vi "Ephys.vi"() -> ()   [LabVIEW 2014]
uses:
  Electrophysiology/Electrophysiology.lvclass
  IntanElectrophysiology/IntanElectrophysiology.lvclass
  IntanElectrophysiology/IntanElectrophysiology.lvclass/IntanElectrophysiology.ctl
panel:
  in  "Base Path For Intan Task Files":path=path "c:/IntanTasks"
  in  "Intan Task":u16(ring)
  in  "Start":bool
  out "Stopped":bool
  in  "Link":bool
  in  "Audio":cluster{"Left":u16, "Right":u16} {"Right" items=["Electrode01"=0, "Electrode02"=1, "Electrode03"=2, "Electrode04"=3, "Electrode05"=4, "Electrode06"=5, "Electrode07"=6, "Electrode08"=7, "Electrode09"=8, "Electrode10"=9, "Electrode11"=10, "Electrode12"=11, "Electrode13"=12, "Electrode14"=13, "Electrode15"=14, "Electrode16"=15, "Electrode17"=16, "Electrode18"=17, "Electrode19"=18, "Electrode20"=19, "Electrode21"=20, "Electrode22"=21, "Electrode23"=22, "Electrode24"=23, "Electrode25"=24, "Electrode26"=25, "Electrode27"=26, "Electrode28"=27, "Electrode29"=28, "Electrode30"=29, "Electrode31"=30, "Electrode32"=31, "Electrode33"=32, "Electrode34"=33, "Electrode35"=34, "Electrode36"=35, "Electrode37"=36, "Electrode38"=37, "Electrode39"=38, "Electrode40"=39, "Electrode41"=40, "Electrode42"=41, "Electrode43"=42, "Electrode44"=43, "Electrode45"=44, "Electrode46"=45, "Electrode47"=46, "Electrode48"=47, "Electrode49"=48, "Electrode50"=49, "Electrode51"=50, "Electrode52"=51, "Electrode53"=52, "Electrode54"=53, "Electrode55"=54, "Electrode56"=55, "Electrode57"=56, "Electrode58"=57, "Electrode59"=58, "Electrode60"=59, "Electrode61"=60, "Electrode62"=61, "Electrode63"=62, "Electrode64"=63, "Electrode65"=64, "Electrode66"=65, "Electrode67"=66, "Electrode68"=67, "Electrode69"=68, "Electrode70"=69, "Electrode71"=70, "Electrode72"=71, "Electrode73"=72, "Electrode74"=73, "Electrode75"=74, "Electrode76"=75, "Electrode77"=76, "Electrode78"=77, "Electrode79"=78, "Electrode80"=79, "Electrode81"=80, "Electrode82"=81, "Electrode83"=82, "Electrode84"=83, "Electrode85"=84, "Electrode86"=85, "Electrode87"=86, "Electrode88"=87, "Electrode89"=88, "Electrode90"=89, "Electrode91"=90, "Electrode92"=91, "Electrode93"=92, "Electrode94"=93, "Electrode95"=94, "Electrode96"=95, "Gnd1"=96, "Gnd2"=97, "Gnd3"=98, "Gnd4"=99, "Photodiode"=102, "Ref1"=100, "Ref2"=101]; "Left" items=["Electrode01"=0, "Electrode02"=1, "Electrode03"=2, "Electrode04"=3, "Electrode05"=4, "Electrode06"=5, "Electrode07"=6, "Electrode08"=7, "Electrode09"=8, "Electrode10"=9, "Electrode11"=10, "Electrode12"=11, "Electrode13"=12, "Electrode14"=13, "Electrode15"=14, "Electrode16"=15, "Electrode17"=16, "Electrode18"=17, "Electrode19"=18, "Electrode20"=19, "Electrode21"=20, "Electrode22"=21, "Electrode23"=22, "Electrode24"=23, "Electrode25"=24, "Electrode26"=25, "Electrode27"=26, "Electrode28"=27, "Electrode29"=28, "Electrode30"=29, "Electrode31"=30, "Electrode32"=31, "Electrode33"=32, "Electrode34"=33, "Electrode35"=34, "Electrode36"=35, "Electrode37"=36, "Electrode38"=37, "Electrode39"=38, "Electrode40"=39, "Electrode41"=40, "Electrode42"=41, "Electrode43"=42, "Electrode44"=43, "Electrode45"=44, "Electrode46"=45, "Electrode47"=46, "Electrode48"=47, "Electrode49"=48, "Electrode50"=49, "Electrode51"=50, "Electrode52"=51, "Electrode53"=52, "Electrode54"=53, "Electrode55"=54, "Electrode56"=55, "Electrode57"=56, "Electrode58"=57, "Electrode59"=58, "Electrode60"=59, "Electrode61"=60, "Electrode62"=61, "Electrode63"=62, "Electrode64"=63, "Electrode65"=64, "Electrode66"=65, "Electrode67"=66, "Electrode68"=67, "Electrode69"=68, "Electrode70"=69, "Electrode71"=70, "Electrode72"=71, "Electrode73"=72, "Electrode74"=73, "Electrode75"=74, "Electrode76"=75, "Electrode77"=76, "Electrode78"=77, "Electrode79"=78, "Electrode80"=79, "Electrode81"=80, "Electrode82"=81, "Electrode83"=82, "Electrode84"=83, "Electrode85"=84, "Electrode86"=85, "Electrode87"=86, "Electrode88"=87, "Electrode89"=88, "Electrode90"=89, "Electrode91"=90, "Electrode92"=91, "Electrode93"=92, "Electrode94"=93, "Electrode95"=94, "Electrode96"=95, "Gnd1"=96, "Gnd2"=97, "Gnd3"=98, "Gnd4"=99, "Photodiode"=102, "Ref1"=100, "Ref2"=101]}
  in  "Volume":dbl(slide)=1.0608183551394462e-08 scale=1e-11..1e-05
  in  "Play":bool
  out "Streaming":bool
  out "Writing Error":bool
  in  "Record":bool=TRUE
  out "Writing Backlog":i32
  in  "NI Recording Task":refnum<k21>="All4498"
  out "MSamples":dbl
  in  "Stop":bool
  # "Audio"
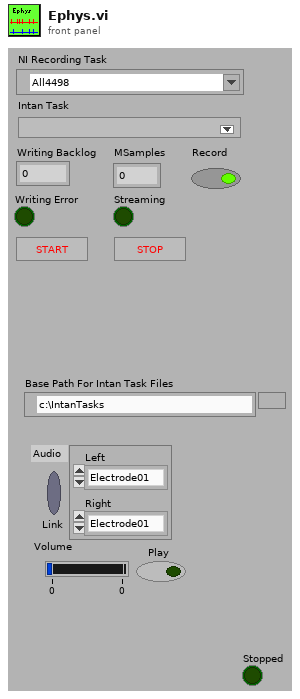
[diagram p1: front panel]
types:
  T1 = enum8{"Enabled", "Disabled", "Disabled and Grayed Out"}
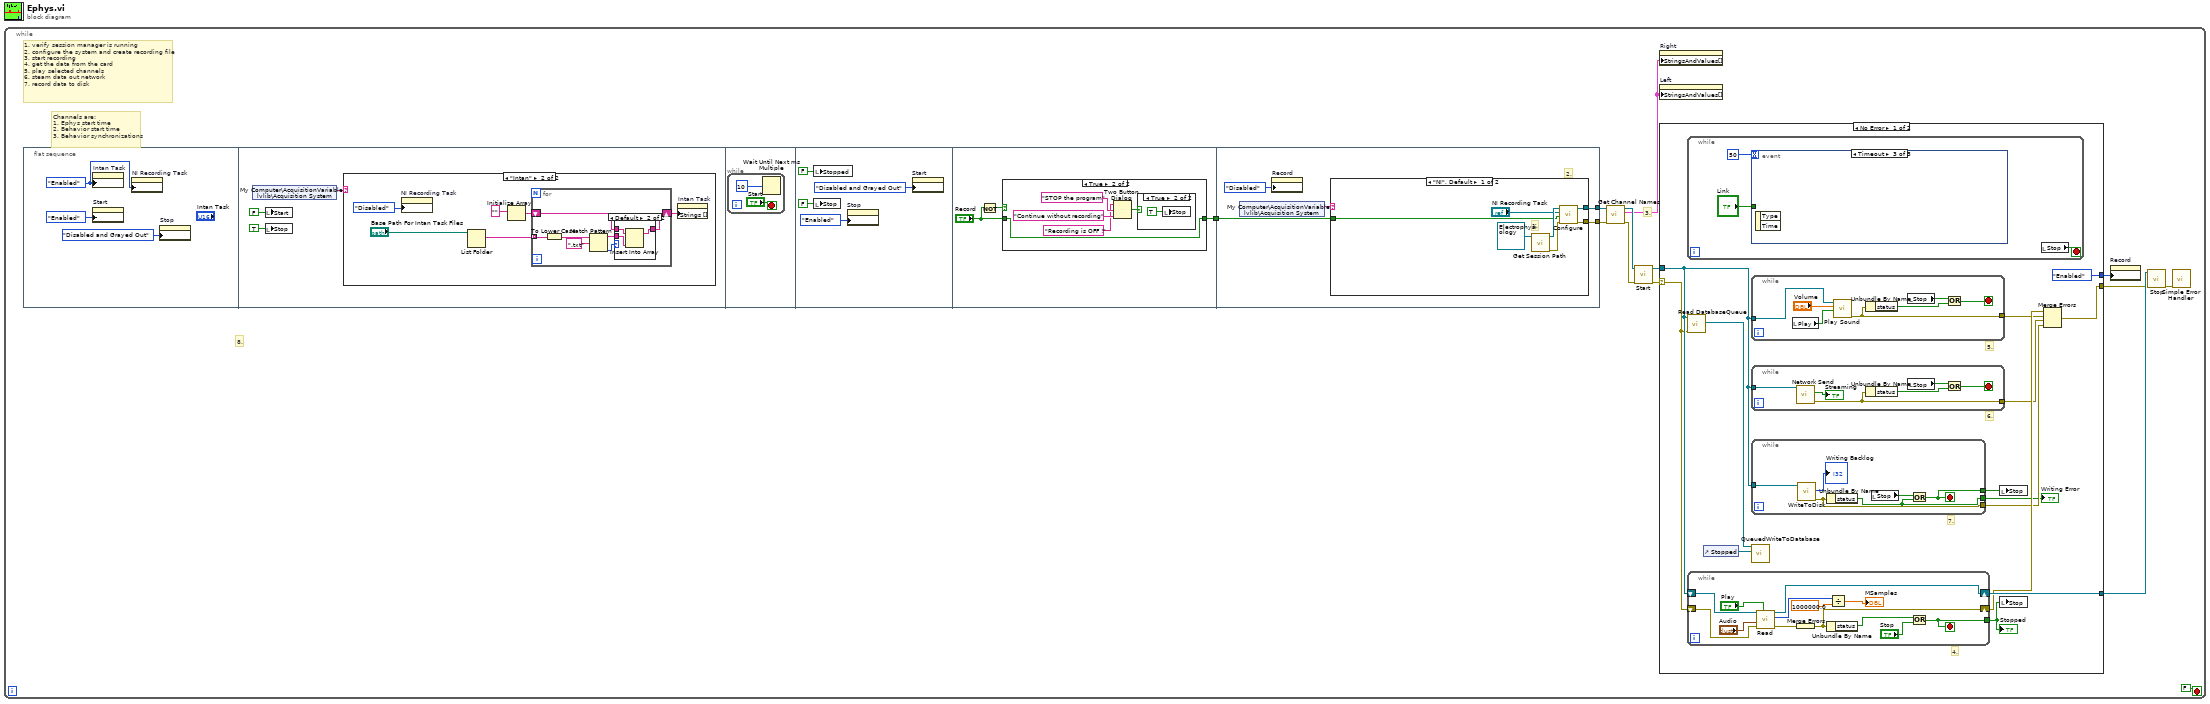
[diagram p0: block diagram]
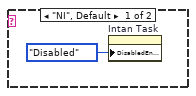
[diagram p2: hidden frame]
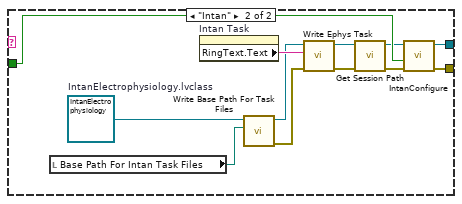
[diagram p6: hidden frame]
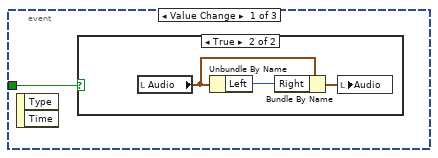
[diagram p7: hidden frame]
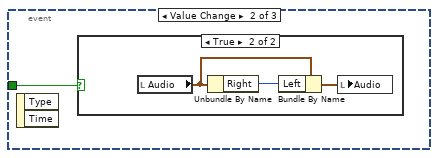
[diagram p9: hidden frame]
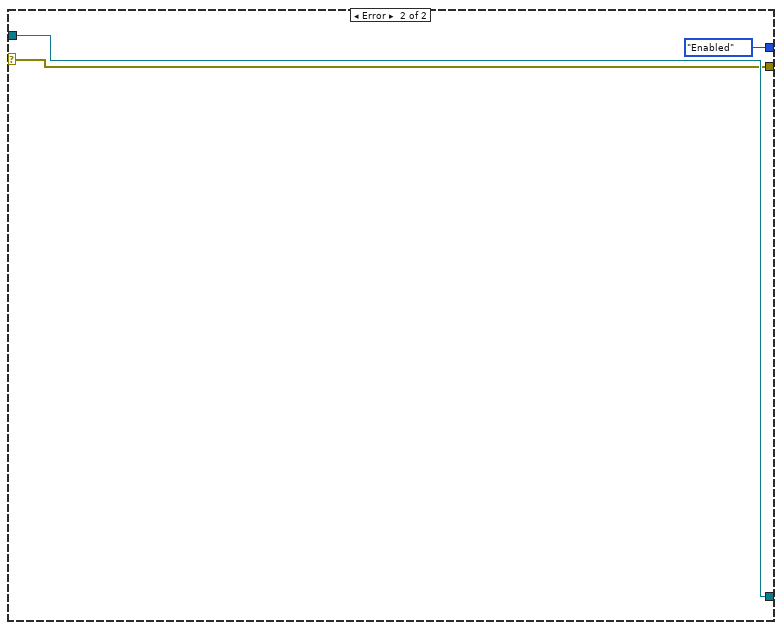
[diagram p11: hidden frame]
diagram:
  n1 = while {
    stop <- FALSE stop-if-true
    # "8."
    # "1. verify session manager is running\n2. configure the system and create recording file\n3. start recording\n4. get the data from the card\n5. play selected channels\n6. steam data out network\n7. record data to disk"
    # "3."
    # "Channels are:\n1. Ephys start time\n2. Behavior start time\n3. Behavior synchronizations"
    n2 = flat-sequence {
      tunnel: [w44] -> w13
      tunnel: [w58] -> w1
      tunnel: w13 -> [w56]
      tunnel: [w55] -> w2
      frame #0 {
        w16 = T1."Enabled" ("Disabled")
        n3 = property on="Intan Task" class="Ring (strict)"("DisabledEnum"=w16) -> ()  [unwired: 2 in, 2 out]
        n4 = property on="Start" class="Bool (strict)"("DisabledEnum"=T1."Enabled" ("Disabled")) -> ()  [unwired: 2 in, 2 out]
        n5 = property on="NI Recording Task" class="DAQmxName (strict)"("DisabledEnum"=w16) -> ()  [unwired: 2 in, 2 out]
        n6 = property on="Stop" class="Bool (strict)"("DisabledEnum"=T1."Disabled and Grayed Out" ("Disabled")) -> ()  [unwired: 2 in, 2 out]
      }
      frame #1 {
        n7 = shared-variable "My Computer\\AcquisitionVariables.lvlib\\Acquisition System"() -> (w17:string)  [unwired: 1 in, 1 out]
        n8 = local write "Start"(FALSE ("Start")) -> ()
        n9 = local write "Stop"(TRUE ("Stop")) -> ()
        n10 = case shown="\"Intan\"" w17 {
          frame "NI", Default {
            n11 = property on="Intan Task" class="Ring (strict)"("DisabledEnum"=T1."Disabled" ("Disabled")) -> ()  [unwired: 2 in, 2 out]
          }
          frame "Intan" {
            n12 = property on="NI Recording Task" class="DAQmxName (strict)"("DisabledEnum"=T1."Disabled" ("Disabled")) -> ()  [unwired: 2 in, 2 out]
            n13 = List Folder(path="Base Path For Intan Task Files") -> (filenames=w24:string[])  [unwired: 3 in, 3 out]
            n14 = Initialize Array("") -> (w22:string[])  [unwired: 1 in]
            n15 = for {
              tunnel: w24 -> [w33] mode=indexing
              shift-right: [w29] -> w21
              shift-left: w22 -> [w28]
              n16 = To Lower Case(string=w33) -> (all lower case string=w32:string)
              n17 = Match Pattern(string=w32, regular expression=".txt") -> (before substring=w27:string, offset past match=w30:i32)  [unwired: 1 in, 2 out]
              n18 = case shown="Default" w30 {
                tunnel: w28 -> [w34 w37]
                tunnel: [w34 w36] -> w29
                tunnel: w27 -> [_ w35]
                frame -1 {
                }
                frame Default {
                  n19 = Insert Into Array(array=w37, new element=w35) -> (w36:string[])  [unwired: 1 in]
                }
              }
            }
            n20 = property on="Intan Task" class="Ring (strict)"("Strings []"=w21) -> ()  [unwired: 2 in, 2 out]
          }
        }
      }
      frame #2 {
        n21 = while {
          stop <- "Start" stop-if-true
          n22 = Wait Until Next ms Multiple(millisecond multiple=u32 10) -> ()  [unwired: 1 out]
        }
      }
      frame #3 {
        n23 = local write "Stopped"(FALSE ("Stopped")) -> ()
        n24 = local write "Stop"(FALSE ("stop")) -> ()
        n25 = property on="Stop" class="Bool (strict)"("DisabledEnum"=T1."Enabled" ("Disabled")) -> ()  [unwired: 2 in, 2 out]
        n26 = property on="Start" class="Bool (strict)"("DisabledEnum"=T1."Disabled and Grayed Out" ("Disabled")) -> ()  [unwired: 2 in, 2 out]
      }
      frame #4 {
        n27 = Not(x="Record") -> (.not. x?=w46:bool)
        n28 = case shown="True" w46 {
          tunnel: "Record" -> [w47 w49]
          tunnel: [w47 w49] -> w44
          frame False {
          }
          frame True {
            n29 = Two Button Dialog(message="Recording is OFF !", 1:"Continue without recording" ("T button name (\"OK\")"), 2:"STOP the program" ("F button name (\"Cancel\")")) -> (T button?=w48:bool)
            n30 = case shown="True" w48 {
              frame False {
              }
              frame True {
                n31 = local write "Stop"(TRUE ("Stop")) -> ()
              }
            }
          }
        }
      }
      frame #5 {
        # "2."
        n32 = shared-variable "My Computer\\AcquisitionVariables.lvlib\\Acquisition System"() -> (w54:string)  [unwired: 1 in, 1 out]
        n33 = property on="Record" class="Bool (strict)"("DisabledEnum"=T1."Disabled" ("Disabled")) -> ()  [unwired: 2 in, 2 out]
        n34 = case shown="\"NI\", Default" w54 {
          tunnel: [w60 w75] -> w58
          tunnel: w56 -> [w62 w76]
          tunnel: [w59 w77] -> w55
          frame "NI", Default {
            # "1."
            n35 = call-dynamic "Get Session Path.vi"("AcquistionObject in"=refnum<class "Electrophysiology.lvclass"> refnum ("Electrophysiology.lvclass")) -> ("error out"=w61:errorcluster, "AcquistionObject out"=w64:refnum<class "Electrophysiology.lvclass">)  [unwired: 8 in, 1 out]
            n36 = call-dynamic "Configure.vi"("error in (no error)"=w61, "Record"=w62, "Recording Channels"="NI Recording Task", "Electrophysiology in"=w64) -> ("error out"=w60:errorcluster, "Electrophysiology out"=w59:refnum<class "Electrophysiology.lvclass">)  [unwired: 6 in]
          }
          frame "Intan" {
            w69 = refnum<class "IntanElectrophysiology.lvclass"> refnum  # IntanElectrophysiology.lvclass
            n37 = local read "Base Path For Intan Task Files"() -> (w68:path)
            n38 = property on="Intan Task" class="Ring (strict)"() -> ("RingText.Text"=w72:string)  [unwired: 2 in, 2 out]
            n39 = call "Write Base Path For Task Files.vi"("Base Path For Task Files"=w68, "IntanElectrophysiology in"=w69) -> ("error out"=w66:errorcluster, "IntanElectrophysiology out"=w67:refnum<class "IntanElectrophysiology.lvclass">)  [unwired: 8 in]
            n40 = call "Write Ephys Task.vi"("error in (no error)"=w66, "Ephys Task"=w72, "IntanElectrophysiology in"=w67) -> ("error out"=w70:errorcluster, "IntanElectrophysiology out"=w71:refnum<class "IntanElectrophysiology.lvclass">)  [unwired: 7 in]
            n41 = call-dynamic "Get Session Path.vi"("error in (no error)"=w70, "AcquistionObject in"=w71) -> ("error out"=w73:errorcluster, "AcquistionObject out"=w74:refnum<class "IntanElectrophysiology.lvclass">)  [unwired: 7 in, 1 out]
            n42 = call "IntanConfigure.vi"("error in (no error)"=w73, "Record"=w76, "IntanElectrophysiology.in"=w74) -> ("error out"=w75:errorcluster, "IntanElectrophysiology.out"=w77:refnum<class "IntanElectrophysiology.lvclass">)  [unwired: 7 in]
          }
        }
      }
    }
    n43 = call-dynamic "Get Channel Names.vi"("error in (no error)"=w1, "Electrophysiology in"=w2) -> ("error out"=w9:errorcluster, "Strings and Numbers"=w8:cluster{refnum<k21>, i32}[], "Electrophysiology out"=w10:refnum<class "Electrophysiology.lvclass">)  [unwired: 7 in]
    n44 = call-dynamic "Start.vi"("error in (no error)"=w9, "Electrophysiology in"=w10) -> ("error out"=w5:errorcluster, "Electrophysiology out"=w4:refnum<class "Electrophysiology.lvclass">)  [unwired: 8 in]
    n45 = property on="Right" class="Ring (strict)"("StringsAndValues[]"=w8) -> ()  [unwired: 2 in, 2 out]
    n46 = property on="Left" class="Ring (strict)"("StringsAndValues[]"=w8) -> ()  [unwired: 2 in, 2 out]
    n47 = case shown="No Error" w5 {
      selector: w5 -> [w78 w136]
      tunnel: w4 -> [w79 w137]
      tunnel: [w91 w137] -> w12
      tunnel: [w87 w136] -> w6
      tunnel: [T1."Enabled" ("Disabled") T1."Enabled" ("Disabled")] -> w7
      frame No Error {
        # "6."
        # "5."
        # "7."
        # "4."
        n48 = while {
          stop <- w94 stop-if-true
          n49 = event shown="[2] Timeout" {
            selector: _ -> [_ _ _]
            dyn-events: _ -> [_ _ _]
            timeout: 50 -> [_ _ _]
            tunnel: "Link" -> [w95 w99 _]
            event "Audio.Left": Value Change {
              n50 = event-data() -> ()  [unwired: 1 in, 2 out]
              n51 = case shown="True" w95 {
                frame False {
                }
                frame True {
                  n52 = local read "Audio"() -> (w98:cluster{"Left":u16, "Right":u16})
                  n53 = Unbundle By Name(w98) -> ("Left"=w97:u16)
                  n54 = Bundle By Name(cluster=w98, "Right"=w97) -> (w96:cluster{"Left":u16, "Right":u16})
                  n55 = local write "Audio"(w96) -> ()
                }
              }
            }
            event "Audio.Right": Value Change {
              n56 = event-data() -> ()  [unwired: 1 in, 2 out]
              n57 = case shown="True" w99 {
                frame False {
                }
                frame True {
                  n58 = local read "Audio"() -> (w102:cluster{"Left":u16, "Right":u16})
                  n59 = Unbundle By Name(w102) -> ("Right"=w101:u16)
                  n60 = Bundle By Name(cluster=w102, "Left"=w101) -> (w100:cluster{"Left":u16, "Right":u16})
                  n61 = local write "Audio"(w100) -> ()
                }
              }
            }
            event Timeout {
              n62 = event-data() -> ()  [unwired: 1 in, 2 out]
            }
          }
          n63 = local read "Stop"() -> (w94:bool)
        }
        n64 = call-dynamic "Read DatabaseQueue.vi"("error in (no error)"=w78, "AcquistionObject in"=w79) -> ("DatabaseQueue"=w81:refnum<queue>)  [unwired: 7 in, 2 out]
        n65 = while {
          tunnel: [w123] -> w82
          shift-right: [w124] -> w90
          shift-left: w78 -> [w122]
          shift-right: [w133] -> w91
          shift-left: w79 -> [w134]
          stop <- w123 stop-if-true
          n66 = call-dynamic "Read.vi"("Enable Sound"="Play", "error in (no error)"=w122, "Audio Channels"="Audio", "Electrophysiology in"=w134) -> ("error out"=w132:errorcluster, "Samples"=w127:u32, "Electrophysiology out"=w133:refnum<class "Electrophysiology.lvclass">)  [unwired: 5 in]
          n67 = Merge Errors(w132) -> (w124:errorcluster)
          n68 = Unbundle By Name(w124) -> ("status"=w131:bool)
          n69 = Divide(x=w127, y=1000000.0) -> (x/y=→"MSamples":dbl)
          n70 = Or(x=w131, y="Stop") -> (x .or. y?=w123:bool)
        }
        "Stopped" <- w82
        n71 = control-ref of="Stopped"() -> (w80:refnum<vi>)
        n72 = while {
          tunnel: w79 -> [w115]
          tunnel: [w109] -> w89
          stop <- w112 stop-if-true
          n73 = local read "Play"() -> (w110:bool)
          n74 = call-dynamic "Play Sound.vi"("Enable Sound"=w110, "Volume"="Volume", "Electrophysiology in"=w115) -> ("error out"=w109:errorcluster)  [unwired: 7 in, 1 out]
          n75 = Unbundle By Name(w109) -> ("status"=w113:bool)
          n76 = local read "Stop"() -> (w114:bool)
          n77 = Or(x=w114, y=w113) -> (x .or. y?=w112:bool)
        }
        n78 = while {
          tunnel: w79 -> [w108]
          tunnel: [w104] -> w88
          stop <- w105 stop-if-true
          n79 = call-dynamic "Network Send.vi"("Electrophysiology in"=w108) -> ("error out"=w104:errorcluster, "Connected"=→"Streaming":bool)  [unwired: 8 in, 1 out]
          n80 = Unbundle By Name(w104) -> ("status"=w106:bool)
          n81 = local read "Stop"() -> (w107:bool)
          n82 = Or(x=w107, y=w106) -> (x .or. y?=w105:bool)
        }
        n83 = while {
          tunnel: w79 -> [w121]
          tunnel: [w118] -> w86
          tunnel: [w117] -> w85
          tunnel: [w116] -> w84
          stop <- w116 stop-if-true
          n84 = call "WriteToDisk.vi"("Electrophysiology.lvclass"=w121) -> ("error out"=w118:errorcluster, "Writing Backlog"=→"Writing Backlog":i32)  [unwired: 8 in, 1 out]
          n85 = Unbundle By Name(w118) -> ("status"=w117:bool)
          n86 = local read "Stop"() -> (w120:bool)
          n87 = Or(x=w120, y=w117) -> (x .or. y?=w116:bool)
        }
        "Writing Error" <- w85
        n88 = call "QueuedWriteToDatabase.vi"("Stop Flag Reference"=w80, "queue"=w81) -> ()  [unwired: 9 in, 1 out]
        n89 = local write "Stop"(w84) -> ()
        n90 = local write "Stop"(w82) -> ()
        n91 = Merge Errors(w90, w89, w88, w86) -> (w87:errorcluster)
      }
      frame Error {
      }
    }
    n92 = property on="Record" class="Bool (strict)"("DisabledEnum"=w7) -> ()  [unwired: 2 in, 2 out]
    n93 = call-dynamic "Stop.vi"("error in (no error)"=w6, "Electrophysiology in"=w12) -> ("error out"=w11:errorcluster)  [unwired: 8 in, 1 out]
    n94 = call <vilib>:"Simple Error Handler.vi"("error in (no error)"=w11) -> ()  [unwired: 4 in, 5 out]
  }
